vi "runDetectionTrt.vi"(8 "error in (no error)":errorcluster, 11 "dl in":refnum<class "dl.lvclass">) -> (0 "error out":errorcluster, 2 "detectionSucc":i32, 3 "dl out":refnum<class "dl.lvclass">)   [LabVIEW 2025, in "dl.lvlib" / "dl.lvclass"]
uses:
  dl.lvclass
  dl.lvclass/dl.ctl
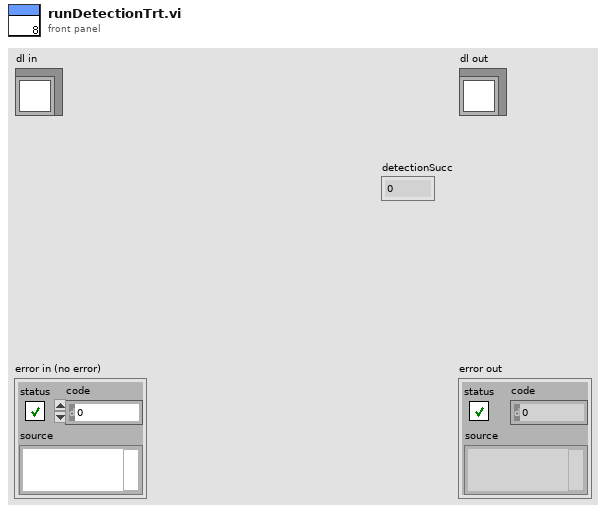
[diagram p1: front panel]
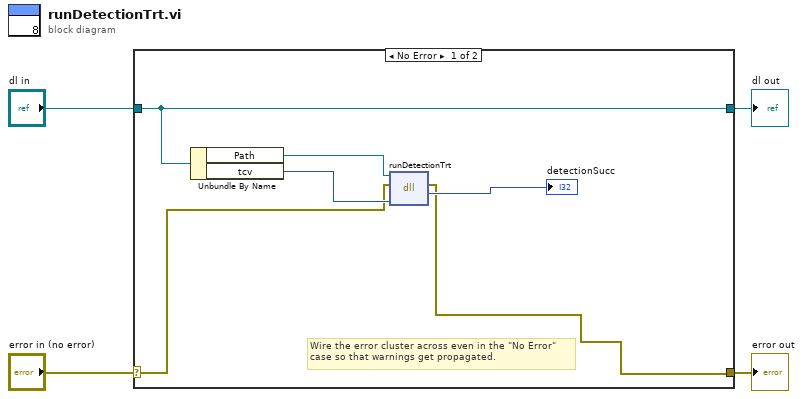
[diagram p0: block diagram]
diagram:
  n1 = case shown="No Error" "error in (no error)" {
    selector: "error in (no error)" -> [w6 w12]
    tunnel: [w5 w12] -> w3
    tunnel: [w10 w11] -> w1
    tunnel: "dl in" -> [w10 w11]
    frame No Error {
      # "Wire the error cluster across even in the \"No Error\"\ncase so that warnings get propagated."
      n2 = Unbundle By Name(w10) -> ("Path"=w9:path, "tcv"=w8:u64)
      n3 = dll-call lib="D:/Test/adslvPackageDev/Resources/TCV_Lib.dll" fn="runDetectionTrt"(path in=w9, error in=w6, "tcv"=w8) -> (error out=w5:errorcluster, "detectionSucc"=→"detectionSucc":i32)  [unwired: 2 in, 1 out]
    }
    frame Error {
    }
  }
  "error out" <- w3
  "dl out" <- w1
